vi "读取任务列表.vi"(8 "error in (no error)":errorcluster caption="错误输入（无错误）", 11 "Cleaningcycle 输入":refnum<class "Cleaning cycle.lvclass">) -> (0 "error out":errorcluster caption="错误输出", 2 "输出簇":cluster{"启用":bool, T1[]}, 3 "Cleaningcycle 输出":refnum<class "Cleaning cycle.lvclass">)   [LabVIEW 2022 SP3, in "Cleaning cycle.lvclass"]
uses:
  Cleaning cycle.lvclass
  Cleaning cycle.lvclass/Cleaning cycle.ctl
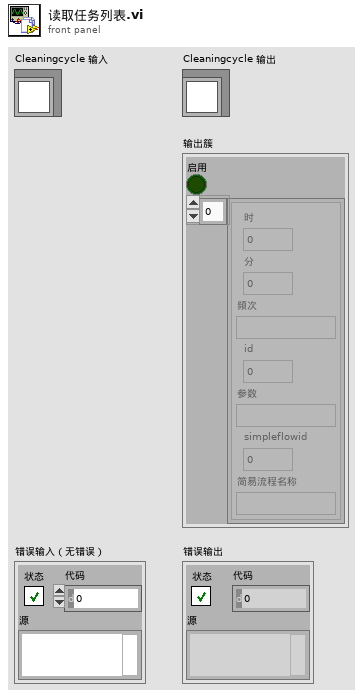
[diagram p1: front panel]
types:
  T1 = typedef "Cleaning cycle.lvclass/周期项.ctl" = cluster{"时":i32, "分":i32, "频次":string, "id":i32, "参数":string, "simpleflowid":i32, "简易流程名称":string}
  T2 = typedef "Cleaning cycle.lvclass/State Data.ctl" = cluster{"配置文件路径":path, "简易流程路径":path, "参数列表":cluster{"String":string, "Value":u16}[], "简易流程列表":cluster{"String":string, "Value":u16}[], "配置信息":T3, "命令":cluster{"触发":bool, "周期项":T1}[]}
  T3 = typedef "Cleaning cycle.lvclass/配置信息.ctl" = cluster{"任务列表":T4}
  T4 = typedef "Cleaning cycle.lvclass/任务.ctl" = cluster{"启用":bool, "项":string[][]}
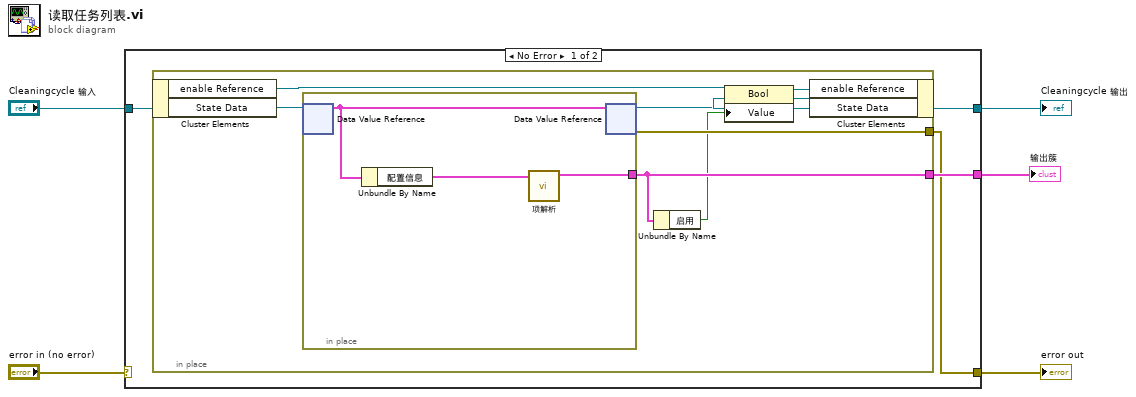
[diagram p0: block diagram]
diagram:
  n1 = case shown="No Error" "error in (no error)" {
    selector: "error in (no error)" -> [_ w21]
    tunnel: [w6 w21] -> w4
    tunnel: [w8 w20] -> w2
    tunnel: "Cleaningcycle 输入" -> [w9 w20]
    tunnel: [w7 _] -> w1
    frame No Error {
      n2 = in-place {
        in-place-border: [w13] -> w7
        in-place-border: [w14] -> w6
        n3 = in-place-cluster #1(w9) -> ("enable Reference"=w12:refnum<vi>, "State Data"=w16:refnum<data-value>)
        n4 = in-place {
          in-place-border: [w19] -> w13
          n5 = in-place-dvr #2(w16) -> (w18:T2)  [unwired: 1 out]
          n6 = Unbundle By Name(w18) -> ("配置信息"=w17:T3)
          n7 = call "项解析.vi"("配置信息"=w17) -> ("任务列表解析"=w19:cluster{"启用":bool, "任务":T1[]})  [unwired: 10 in]
          n8 = in-place-dvr #2(w18) -> (w15:refnum<data-value>, w14:errorcluster)
        }
        n9 = Unbundle By Name(w13) -> ("启用"=w10:bool)
        n10 = property class="Bool"(reference=w12, "Value"=w10) -> (reference out=w11:refnum<vi>)  [unwired: 1 in, 1 out]
        n11 = in-place-cluster #1("enable Reference"=w11, "State Data"=w15) -> (w8:refnum<class "Cleaning cycle.lvclass">)
      }
    }
    frame Error {
    }
  }
  "error out" <- w4
  "Cleaningcycle 输出" <- w2
  "输出簇" <- w1
